vi "DataReceiver.vi"() -> ()   [LabVIEW 2010]
doc: "This VI in conjunction with Target Fullness.vi demonstrates how to use network streams properties to determine how effectively data is being delivered through the network stream before it becomes congested and has to block before accepting new data. Setting the writer wait time smaller than the reader wait time will cause the reader and writer to gradually fill up. In this situation, the reader is the bottleneck of the transfer. Setting the reader wait time smaller than the writer wait time will cause the reader and writer to gradually empty. In this situation, the writer is the bottleneck of the transfer.\n\n<B>Note:</B> Requires Target Fullnes.vi located in the same directory as this VI."
uses:
  C:/Program Files/National Instruments/LabVIEW 2010/resource/objmgr/ni.dex.rc
panel:
  out "Waveform Chart":waveform(dbl)[](graph)
  out "error out":errorcluster
  in  "Reader Wait Time":u32=25
  in  "stop":bool
  out "Elements in Reader":i32(slide) scale=0.0..100.0
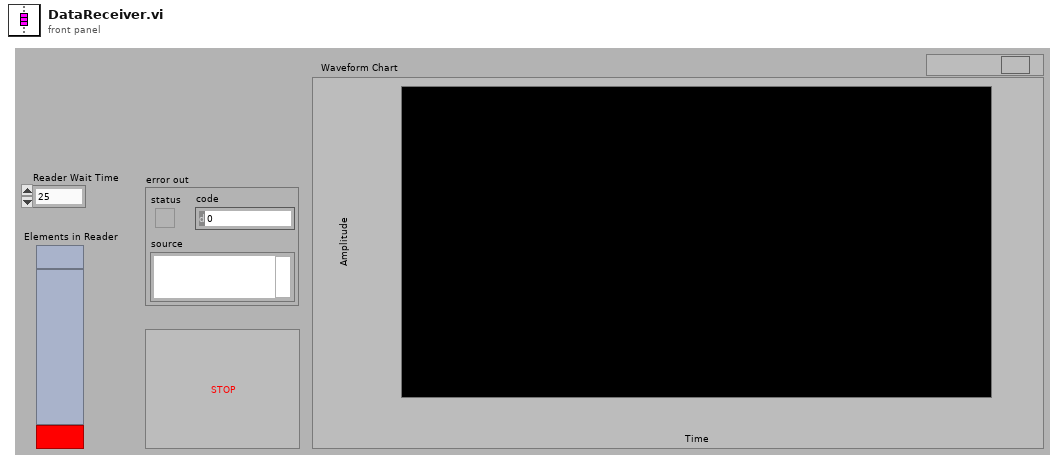
[diagram p1: front panel]
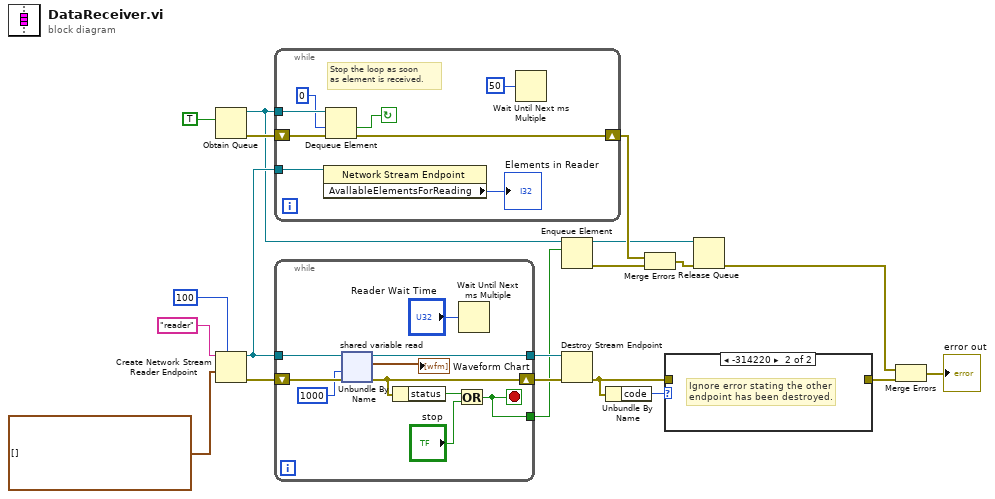
[diagram p0: block diagram]
diagram:
  n1 = Obtain Queue(element data type=TRUE ("stop")) -> (queue out=w8:refnum<queue>, error out=w13:errorcluster)  [unwired: 4 in, 1 out]
  n2 = Create Network Stream Reader Endpoint(7:100 ("reader buffer size"), 9:waveform(dbl)[] [], 11:"reader" ("writer name")) -> (0:w19:errorcluster, 3:w16:refnum<k21>)  [unwired: 3 in]
  n3 = while {
    tunnel: w16 -> [w28]
    tunnel: w8 -> [w25]
    shift-right: [w23] -> w15
    shift-left: w13 -> [w22]
    stop <- w21 continue-if-true
    # "Stop the loop as soon \nas element is received."
    n4 = property class="Network Stream Endpoint"(reference=w28) -> ("AvallableElementsForReading"=→"Elements in Reader":i32)  [unwired: 1 in, 2 out]
    n5 = Dequeue Element(queue=w25, timeout in ms (-1)=0, error in (no error)=w22) -> (timed out?=w21:bool, error out=w23:errorcluster)  [unwired: 2 out]
    n6 = Wait Until Next ms Multiple(millisecond multiple=u32 50 ("milliseconds to wait")) -> ()  [unwired: 1 out]
  }
  n7 = while {
    tunnel: w16 -> [w37]
    tunnel: [w36] -> w18
    shift-right: [w31] -> w17
    shift-left: w19 -> [w38]
    tunnel: [w30] -> w5
    stop <- w30 stop-if-true
    n8 = shared-variable-read(w37, w38, 1000 ("timeout in ms (-1)")) -> (w36:refnum<k21>, w31:errorcluster, →"Waveform Chart":waveform(dbl)[])  [unwired: 1 out]
    n9 = Unbundle By Name(w31) -> ("status"=w32:bool)
    n10 = Or(x=w32, y="stop") -> (x .or. y?=w30:bool)
    n11 = Wait Until Next ms Multiple(millisecond multiple="Reader Wait Time") -> ()  [unwired: 1 out]
  }
  n12 = Enqueue Element(queue=w8, element=w5) -> (queue out=w9:refnum<queue>, error out=w10:errorcluster)  [unwired: 2 in, 1 out]
  n13 = Destroy Stream Endpoint(8:w17, 11:w18) -> (0:w6:errorcluster)
  n14 = Unbundle By Name(w6) -> ("code"=w7:i32)
  n15 = Merge Errors(w15, w10) -> (w12:errorcluster)
  n16 = case shown="-314220" w7 {
    tunnel: w6 -> [w39 _]
    tunnel: [w39 _] -> w4
    frame 0, Default {
    }
    frame -314220 {
      # "Ignore error stating the other\nendpoint has been destroyed."
    }
  }
  n17 = Release Queue(queue=w9, error in (no error)=w12) -> (error out=w3:errorcluster)  [unwired: 1 in, 2 out]
  n18 = Merge Errors(w3, w4) -> (→"error out":errorcluster)
